vi "User_Current_Read.vi"(8 "error in (no error)":errorcluster caption="错误输入（无错误）", 11 "Name":string) -> (0 "error out":errorcluster caption="错误输出", 3 "User_Info":T1 {"User_Right" items=["管理员", "操作员"]})   [LabVIEW 2020]
uses:
  User_Manage/User_Databse/User_Info.ctl
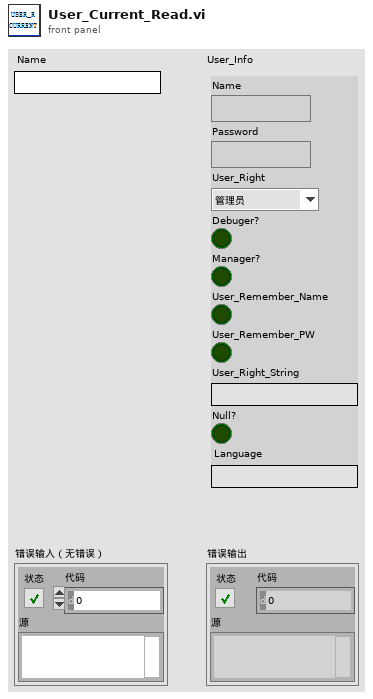
[diagram p1: front panel]
types:
  T1 = typedef "User_Info.ctl" = cluster{"Name":string, "Password":string, "User_Right":u16, "Debuger?":bool, "Manager?":bool, "User_Remember_Name":bool, "User_Remember_PW":bool, "User_Right_String":string, "Null?":bool, "Language":string}
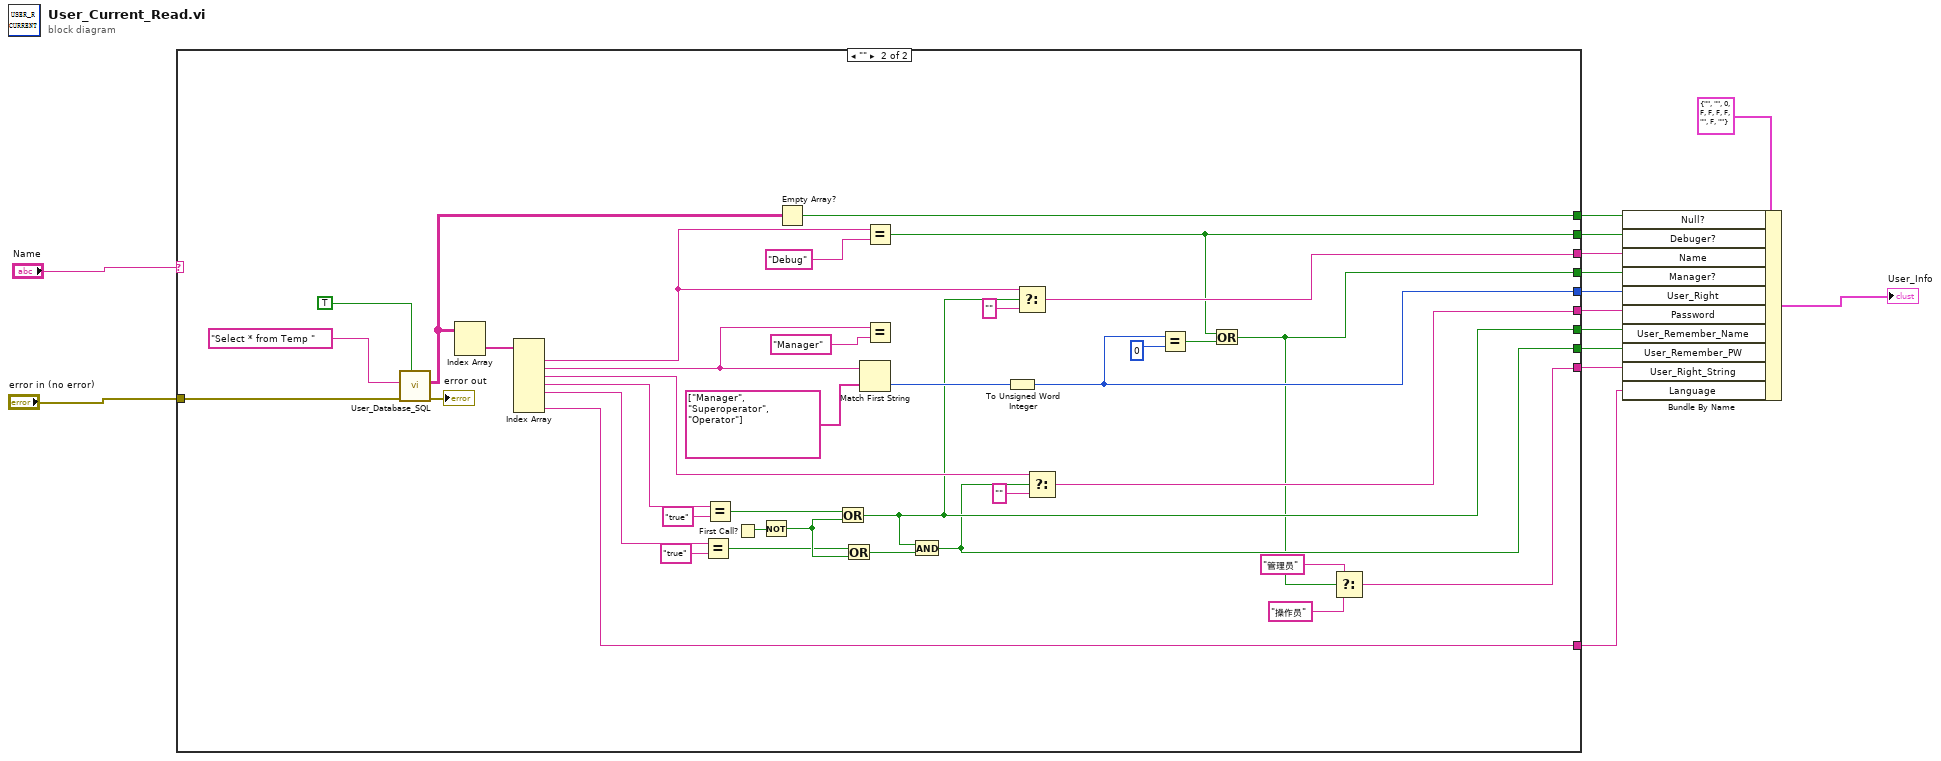
[diagram p0: block diagram]
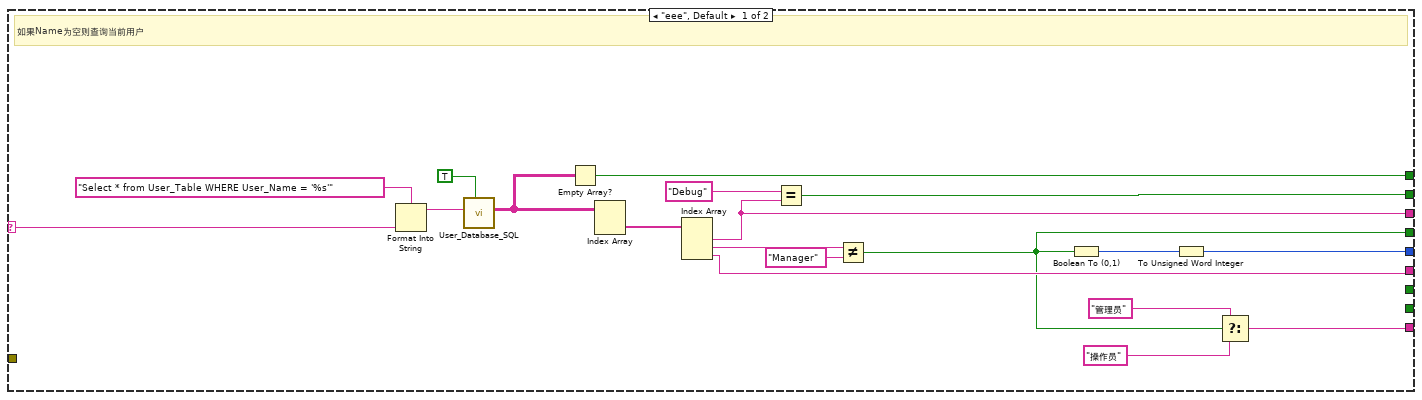
[diagram p2: hidden frame]
diagram:
  n1 = case shown="\"\"" "Name" {
    selector: "Name" -> [w30 _]
    tunnel: "error in (no error)" -> [_ w66]
    tunnel: [w27 w36] -> w13
    tunnel: [w26 w43] -> w12
    tunnel: [w18 w35] -> w11
    tunnel: [w21 w53] -> w10
    tunnel: [_ w40] -> w9
    tunnel: [_ w38] -> w8
    tunnel: [w22 w42] -> w5
    tunnel: [w17 w41] -> w4
    tunnel: [w15 w44] -> w2
    tunnel: [_ w34] -> w1
    frame "eee", Default {
      # "如果Name为空则查询当前用户"
      n2 = Format Into String(format string="Select * from User_Table WHERE User_Name = '%s'" ("SQL query"), w30) -> (resulting string=w33:string)  [unwired: 2 in, 1 out]
      n3 = call "User_Database_SQL.vi"("Get Record"=TRUE, "SQL query"=w33) -> ("Record"=w16:string[][])  [unwired: 7 in, 2 out]
      n4 = Empty Array?(array=w16) -> (empty?=w15:bool)
      n5 = Index Array(array=w16) -> (element=w29:string[])  [unwired: 2 in]
      n6 = Index Array(array=w29) -> (element #1=w26:string, element #2=w25:string, element #3=w21:string)  [unwired: 3 in]
      n7 = Equal?(x="Debug", y=w26) -> (x = y?=w27:bool)
      n8 = Not Equal?(x=w25, y="Manager") -> (x != y?=w18:bool)
      n9 = Boolean To (0,1)(Boolean=w18) -> (0, 1=w23:i16)
      n10 = To Unsigned Word Integer(number=w23) -> (unsigned 16bit integer=w22:u16)
      n11 = Select(t="管理员", s=w18, f="操作员") -> (s? t:f=w17:string)
    }
    frame "" {
      n12 = call "User_Database_SQL.vi"("Get Record"=TRUE, "error in (no error)"=w66, "SQL query"="Select * from Temp ") -> ("error out"=→"error out":errorcluster, "Record"=w49:string[][])  [unwired: 6 in, 1 out]
      n13 = Index Array(array=w49) -> (element=w69:string[])  [unwired: 2 in]
      n14 = Index Array(array=w69) -> (element #1=w56:string, element #2=w63:string, element #3=w54:string, element #4=w61:string, element #5=w58:string, element #7=w34:string)  [unwired: 7 in, 1 out]
      n15 = Equal?(x=w58, y="true") -> (x = y?=w45:bool)
      n16 = Equal?(x=w61, y="true") -> (x = y?=w47:bool)
      n17 = First Call?() -> (First Call?: T/F=w48:bool)
      n18 = Not(x=w48) -> (.not. x?=w46:bool)
      n19 = Empty Array?(array=w49) -> (empty?=w44:bool)
      n20 = Or(x=w47, y=w46) -> (x .or. y?=w40:bool)
      n21 = Or(x=w45, y=w46) -> (x .or. y?=w39:bool)
      n22 = Match First String(2:string[] ["Manager", "Superoperator", "Operator"] ("字符串数组"), 3:w63) -> (0:w62:i32)  [unwired: 1 out]
      n23 = Equal?(x=w56, y="Debug") -> (x = y?=w36:bool)
      n24 = Equal?(x=w63, y="Manager") -> ()  [unwired: 1 out]
      n25 = And(x=w40, y=w39) -> (x .and. y?=w38:bool)
      n26 = To Unsigned Word Integer(number=w62) -> (unsigned 16bit integer=w42:u16)
      n27 = Select(t=w56, s=w40, f="") -> (s? t:f=w43:string)
      n28 = Select(t=w54, s=w38, f="") -> (s? t:f=w53:string)
      n29 = Equal?(x=w42, y=u16 0) -> (x = y?=w37:bool)
      n30 = Or(x=w36, y=w37) -> (x .or. y?=w35:bool)
      n31 = Select(t="管理员", s=w35, f="操作员") -> (s? t:f=w41:string)
    }
  }
  n32 = Bundle By Name(cluster=T1 {"Name"="", "Password"="", "User_Right"=0, "Debuger?"=FALSE, "Manager?"=FALSE, "User_Remember_Name"=FALSE, "User_Remember_PW"=FALSE, "User_Right_String"="", "Null?"=FALSE, "Language"=""} ("簇"), "Null?"=w2, "Debuger?"=w13, "Name"=w12, "Manager?"=w11, "User_Right"=w5, "Password"=w10, "User_Remember_Name"=w9, "User_Remember_PW"=w8, "User_Right_String"=w4, "Language"=w1) -> (→"User_Info":T1)
